vi "Reset.vi"(0 "VISA resource name":refnum<visa-resource-name>, 11 "error in (no error)":errorcluster) -> (4 "VISA resource name out":refnum<visa-resource-name>, 15 "error out":errorcluster)   [LabVIEW 2020, in "eec EST 300.lvlib"]
doc: "Reset the instrument to <B>original power on configuration</B>. Does not clear Enable register for Standard Summary Status or Standard Event Registers. Does not clear the output queue. Does not clear the power-on-status-clear flag."
uses:
  <instrlib>/eec EST 300/eec EST 300.lvlib
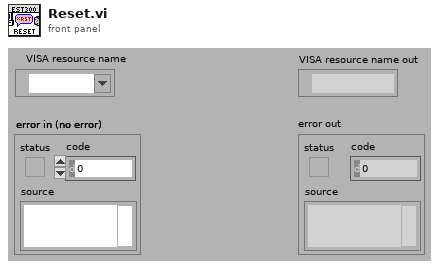
[diagram p1: front panel]
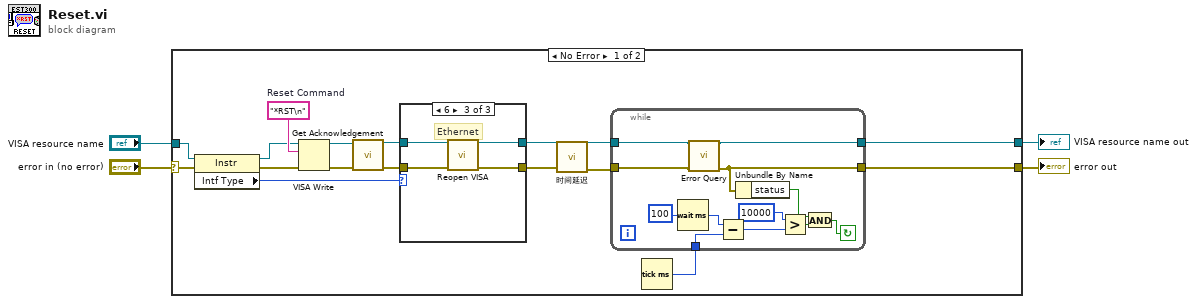
[diagram p0: block diagram]
diagram:
  n1 = case shown="No Error" "error in (no error)" {
    selector: "error in (no error)" -> [w17 w41]
    tunnel: "VISA resource name" -> [w16 w42]
    tunnel: [w5 w42] -> w3
    tunnel: [w6 w41] -> w2
    frame No Error {
      w20 = "*RST\n"  # Reset Command
      n2 = property on="Property Node" class="Instr"(reference=w16, error in=w17) -> (reference out=w15:refnum<visa-resource-name>, error out=w14:errorcluster, "Intf Type"=w13:u16)
      n3 = VISA Write(VISA resource name=w15, write buffer=w20, error in (no error)=w14) -> (VISA resource name out=w18:refnum<visa-resource-name>, error out=w19:errorcluster)  [unwired: 1 out]
      n4 = call <instrlib>:"Get Acknowledgement.vi"("VISA resource name"=w18, "error in (no error)"=w19) -> ("VISA resource name out"=w11:refnum<visa-resource-name>, "error out"=w12:errorcluster)  [unwired: 12 in]
      n5 = case shown="6" w13 {
        tunnel: w12 -> [w34 w36 w39]
        tunnel: [w34 w36 w38] -> w7
        tunnel: w11 -> [w33 w35 w40]
        tunnel: [w33 w35 w37] -> w8
        frame Default {
        }
        frame 1, 4 {
          # "GPIB. Serial"
        }
        frame 6 {
          # "Ethernet"
          n6 = call <instrlib>:"Reopen VISA.vi"("VISA resource name"=w40, "error in (no error)"=w39) -> ("VISA resource name out"=w37:refnum<visa-resource-name>, "error out"=w38:errorcluster)  [unwired: 12 in]
        }
      }
      n7 = call "时间延迟"("error in (no error)"=w7) -> ("error out"=w10:errorcluster)  [unwired: 10 in]
      n8 = Tick Count (ms)() -> (millisecond timer value=w9:u32)
      n9 = while {
        tunnel: [w22] -> w5
        tunnel: [w21] -> w6
        tunnel: w8 -> [w24]
        tunnel: w10 -> [w23]
        tunnel: w9 -> [w31]
        stop <- w26 continue-if-true
        n10 = Wait (ms)(milliseconds to wait=u32 100 ("等待时间（毫秒）")) -> (millisecond timer value=w32:u32)
        n11 = call <instrlib>:"Error Query.vi"("VISA resource name"=w24, "error in (no error)"=w23) -> ("VISA resource name out"=w22:refnum<visa-resource-name>, "error out"=w21:errorcluster)  [unwired: 10 in, 2 out]
        n12 = Subtract(x=w32, y=w31) -> (x-y=w28:u32)
        n13 = Unbundle By Name(w21) -> ("status"=w30:bool)
        n14 = Greater?(x=10000, y=w28) -> (0:w27:bool)
        n15 = And(x=w30, y=w27) -> (x .and. y?=w26:bool)
      }
    }
    frame Error {
    }
  }
  "error out" <- w2
  "VISA resource name out" <- w3
